vi "faultdia.vi"() -> ()   [LabVIEW 2018]
uses:
  <vilib>/Utility/file.llb/Read Delimited Spreadsheet (DBL).vi
panel:
  in  "选项卡控件":enum32{"分类训练", "状态监测", "故障诊断"}(tab)
  in  "隐藏层":dbl[](array[numeric])=[20.0, 20.0, 20.0]
  in  "残差值":dbl=1e-05
  in  "学习率":dbl=0.01
  in  "最大训练次数":dbl=1000.0
  out "训练完毕":bool
  out "导入完毕":bool
  in  "开始训练":bool
  in  "数据导入":bool
  in  "分类标签路径-output":path=path "E:/BIGzuoye2022/faultdig/gogoLabVIEW/faultdig/output.csv"
  in  "特征变量路径-input":path=path "E:/BIGzuoye2022/faultdig/gogoLabVIEW/faultdig/input.csv"
  out "总体分类结果\n Accuracy":dbl[](array[numeric])
  out "内阻偏大故障\n Accuracy":dbl[](array[numeric])
  out "SOC偏小故障\n Accuracy":dbl[](array[numeric])
  out "容量偏小故障\n Accuracy":dbl[](array[numeric])
  out "波形图":dbl[][](graph)
  out "all rows":dbl[][](array[numeric]) caption="特征变量查看"
  out "all rows 2":dbl[][](array[numeric]) caption="分类标签查看"
  in  "验证集-input":path=path "E:/BIGzuoye2022/faultdig/gogoLabVIEW/faultdig/variinput.csv"
  in  "验证集-output":path=path "E:/BIGzuoye2022/faultdig/gogoLabVIEW/faultdig/varioutput.csv"
  in  "继续监测":bool
  out "监测暂停":bool
  out "开始监测":bool
  in  "开始监测":bool
  in  "监测暂停":bool
  out "电压特征1实时监测":T1(graph)
  in  "Cell6连接":bool
  in  "Cell5连接":bool
  in  "Cell4连接":bool
  in  "Cell3连接":bool
  in  "Cell2连接":bool
  in  "Cell1连接":bool
  out "时间序列":dbl
  out "Cell1":dbl[](array[numeric])
  out "Cell2":dbl[](array[numeric])
  out "Cell3":dbl[](array[numeric])
  out "Cell4":dbl[](array[numeric])
  out "Cell5":dbl[](array[numeric])
  out "Cell6":dbl[](array[numeric])
  out "SOC实时监测":T1(graph)
  out "波形图表":T1(graph)
  out "随机生成特征变量":bool
  out "电池实时故障诊断":bool
  in  "电池实时故障诊断":bool
  out "电池监测时序":dbl
  in  "暂停诊断":bool
  in  "随机生成电池信息":bool
  out "电池正常1":bool[](array[boolean])
  out "内阻偏大故障1":bool[](array[boolean])
  out "SOC偏小故障1":bool[](array[boolean])
  out "容量偏小故障1":bool[](array[boolean])
  out "内阻偏大故障2":bool[](array[boolean])
  out "SOC偏小故障2":bool[](array[boolean])
  out "容量偏小故障2":bool[](array[boolean])
  out "电池正常2":bool[](array[boolean])
  out "内阻偏大故障3":bool[](array[boolean])
  out "SOC偏小故障3":bool[](array[boolean])
  out "容量偏小故障3":bool[](array[boolean])
  out "电池正常3":bool[](array[boolean])
  out "内阻偏大故障4":bool[](array[boolean])
  out "SOC偏小故障4":bool[](array[boolean])
  out "容量偏小故障4":bool[](array[boolean])
  out "电池正常4":bool[](array[boolean])
  out "内阻偏大故障5":bool[](array[boolean])
  out "SOC偏小故障5":bool[](array[boolean])
  out "容量偏小故障5":bool[](array[boolean])
  out "电池正常5":bool[](array[boolean])
  out "内阻偏大故障6":bool[](array[boolean])
  out "SOC偏小故障6":bool[](array[boolean])
  out "容量偏小故障6":bool[](array[boolean])
  out "电池正常6":bool[](array[boolean])
  in  "继续诊断":bool
  out "内阻偏大故障_rand":bool[](array[boolean])
  out "SOC偏小故障_rand":bool[](array[boolean])
  out "容量偏小故障_rand":bool[](array[boolean])
  out "电池正常_rand":bool[](array[boolean])
  out "随机生成特征变量 2":dbl[][](array[numeric])
  out "BP实际输出":dbl[][](array[numeric])
  out "诊断结果":dbl[][](array[numeric])
  # "默认：训练次数1000；学习率0.01；残差值0.00001；隐藏层[20,20,20].\n！！运行前修改文件路径！！"
  # "SOC\n\nSOC特征1\n\nSOC特征2\n\nSOC特征3\n\nSOC特征4\n\n电压特征1\n\n电压特征2\n\n电压特征3\n\n电压特征4"
  # "SOC\n\nSOC特征1\n\nSOC特征2\n\nSOC特征3\n\nSOC特征4\n\n电压特征1\n\n电压特征2\n\n电压特征3\n\n电压特征4"
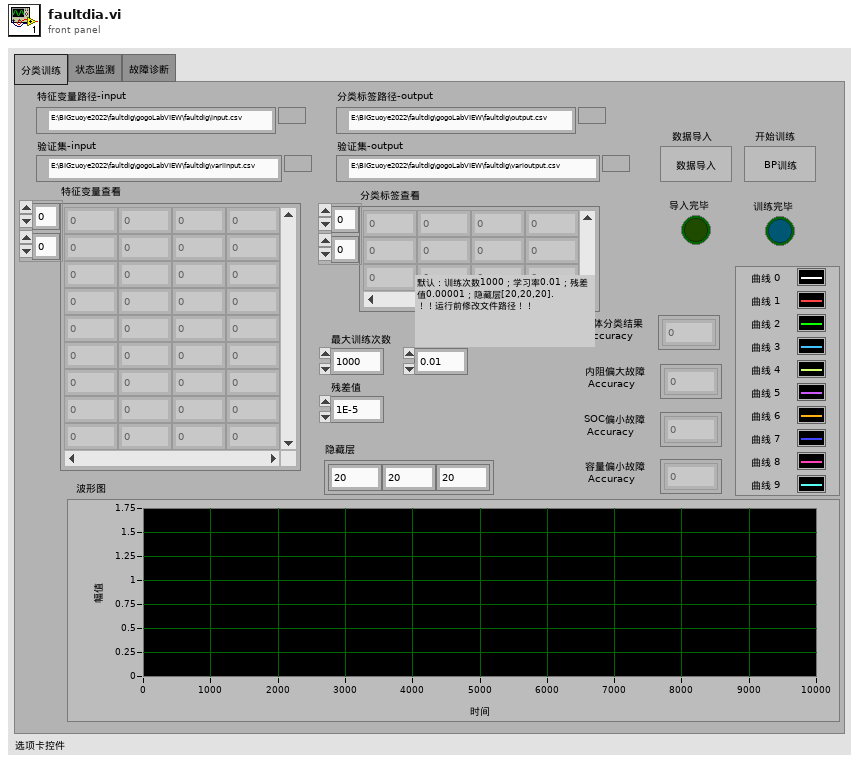
[diagram p1: front panel]
types:
  T1 = cluster{"Numeric":dbl, "Numeric":dbl, "Numeric":dbl, "Numeric":dbl, "Numeric":dbl, "Numeric":dbl}
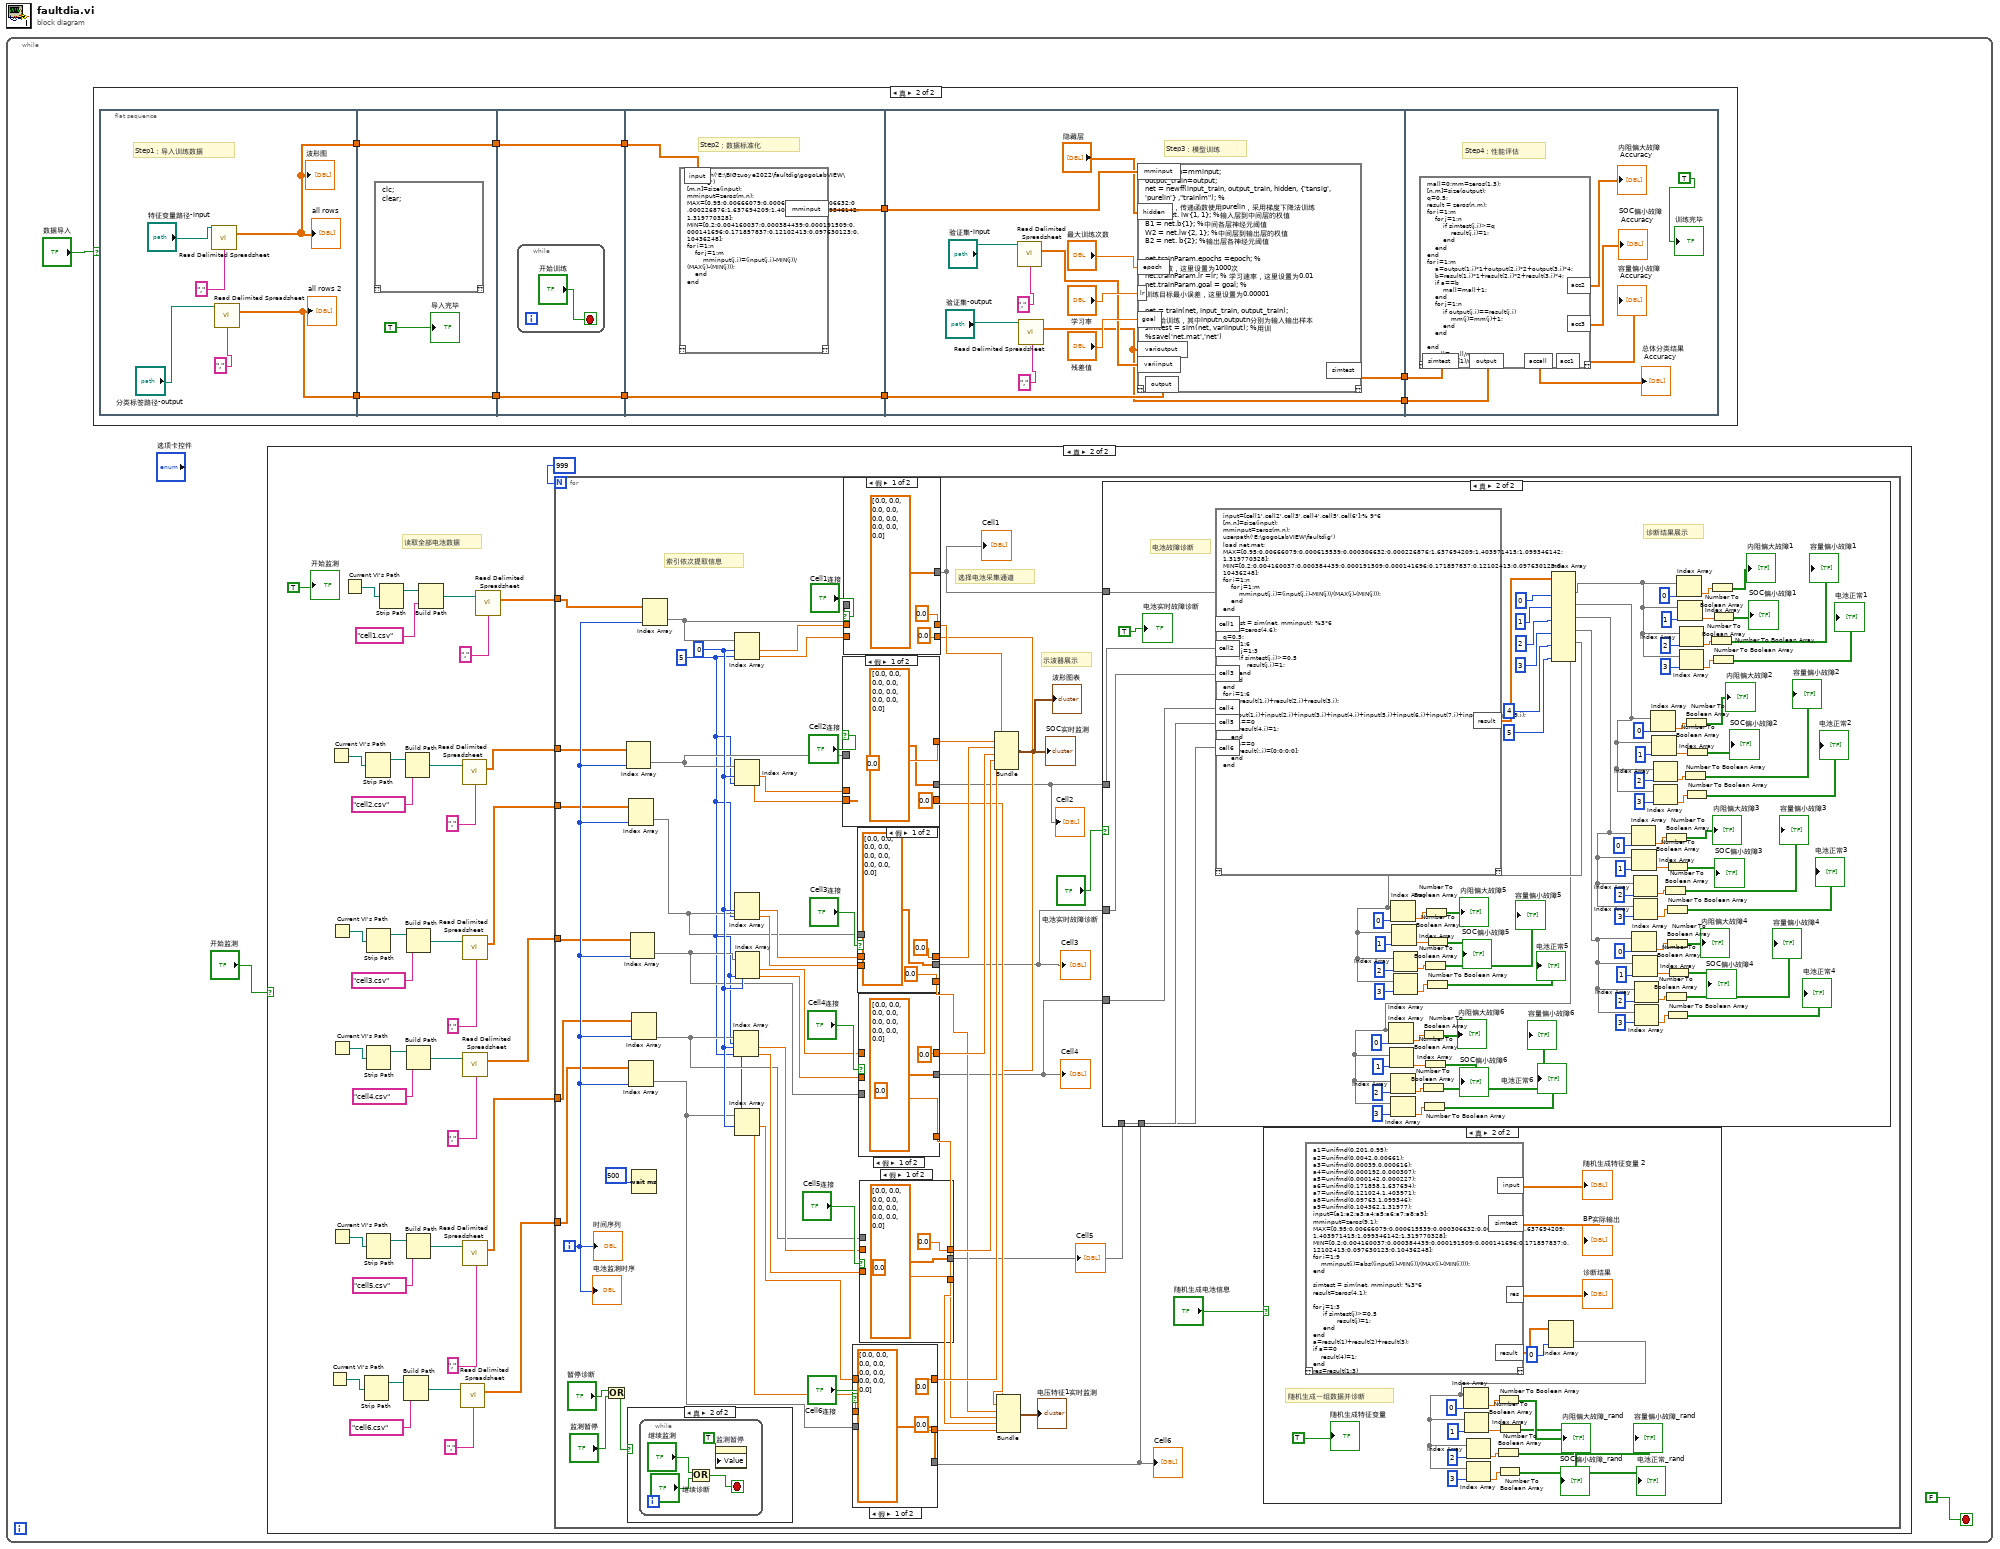
[diagram p0: block diagram]
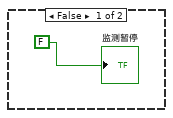
[diagram p11: hidden frame]
diagram:
  n1 = while {
    stop <- FALSE stop-if-true
    n2 = case shown="真" "数据导入" {
      frame False {
      }
      frame True {
        n3 = flat-sequence {
          tunnel: [w266] -> w262
          tunnel: [w265] -> w261
          tunnel: [w271] -> w260
          tunnel: w262 -> [w271]
          tunnel: w261 -> [w270]
          tunnel: [w270] -> w259
          tunnel: w260 -> [w273]
          tunnel: [w273] -> w258
          tunnel: w259 -> [w272]
          tunnel: [w272] -> w257
          tunnel: w258 -> [w277]
          tunnel: [w276] -> w256
          tunnel: [w275] -> w255
          tunnel: w257 -> [w275]
          tunnel: w256 -> [w290]
          tunnel: w255 -> [w288]
          tunnel: [w289] -> w254
          tunnel: [w278] -> w253
          tunnel: w254 -> [w297]
          tunnel: w253 -> [w291]
          frame #0 {
            # "Step1：导入训练数据"
            n4 = call-poly <vilib>:"Read Delimited Spreadsheet.vi"("file path (dialog if empty)"="特征变量路径-input", "delimiter (\\t)"=",") -> ("all rows"=w266:dbl[][])  [unwired: 8 in, 5 out]
            "all rows" <- w266
            "波形图" <- w266
            n5 = call-poly <vilib>:"Read Delimited Spreadsheet.vi"("file path (dialog if empty)"="分类标签路径-output", "delimiter (\\t)"=",") -> ("all rows"=w265:dbl[][])  [unwired: 8 in, 5 out]
            "all rows 2" <- w265
          }
          frame #1 {
            n6 = script code="clc;\nclear;"() -> ()  [unwired: 1 in, 1 out]
            "导入完毕" <- TRUE
          }
          frame #2 {
            n7 = while {
              stop <- "开始训练" stop-if-true
            }
          }
          frame #3 {
            # "Step2：数据标准化"
            n8 = script code="userpath('E:\\BIGzuoye2022\\faultdig\\gogoLabVIEW\\faultdig')\n[m,n]=size(input);\nmminput=zeros(m,n);\nMAX=[0.95;0.00666079;0.000615539;0.000306632;0.000226876;1.637694209;1.403971415;1.099346142;1.319770328];\nMIN=[0.2;0.004160037;0.000384439;0.000191509;0.000141696;0.171857837;0.12102413;0.097630123;0.10436248];\nfor i=1:n\n    for j=1:m\n        mminput(j,i)=(input(j,i)-MIN(j))/(MAX(j)-(MIN(j)));\n    end \nend"("input"=w277) -> ("mminput"=w276:dbl[][])  [unwired: 1 in, 1 out]
          }
          frame #4 {
            # "Step3：模型训练"
            n9 = call-poly <vilib>:"Read Delimited Spreadsheet.vi"("file path (dialog if empty)"="验证集-input", "delimiter (\\t)"=",") -> ("all rows"=w279:dbl[][])  [unwired: 8 in, 5 out]
            n10 = call-poly <vilib>:"Read Delimited Spreadsheet.vi"("file path (dialog if empty)"="验证集-output", "delimiter (\\t)"=",") -> ("all rows"=w278:dbl[][])  [unwired: 8 in, 5 out]
            n11 = script code="input_train=mminput;\noutput_train=output;\nnet = newff(input_train, output_train, hidden, {'tansig', 'purelin'} ,\"trainlm\"); % 建立模型，传递函数使用purelin，采用梯度下降法训练\nW1 = net. iw{1, 1}; %输入层到中间层的权值\nB1 = net.b{1}; %中间各层神经元阈值\nW2 = net.lw{2, 1}; %中间层到输出层的权值\nB2 = net. b{2}; %输出层各神经元阈值\n\nnet.trainParam.epochs =epoch; % 训练次数，这里设置为1000次\nnet.trainParam.lr =lr; % 学习速率，这里设置为0.01\nnet.trainParam.goal = goal; % 训练目标最小误差，这里设置为0.00001\n\nnet = train(net, input_train, output_train); %开始训练，其中inputn,outputn分别为输入输出样本\nsimtest = sim(net, variinput); %用训\n%save('net.mat','net')"("mminput"=w290, "output"=w288, "epoch"="最大训练次数", "lr"="学习率", "goal"="残差值", "hidden"="隐藏层", "varioutput"=w278, "variinput"=w279) -> ("simtest"=w289:dbl[][])  [unwired: 1 in, 1 out]
          }
          frame #5 {
            # "Step4：性能评估"
            n12 = script code="mall=0;mm=zeros(1,3);\n[n,m]=size(output);\nq=0.5;\nresult = zeros(n,m);\nfor i=1:m\n    for j=1:n\n        if simtest(j,i)>=q\n            result(j,i)=1;\n        end\n    end\nend\nfor i=1:m\n    a=output(1,i)*1+output(2,i)*2+output(3,i)*4;\n    b=result(1,i)*1+result(2,i)*2+result(3,i)*4;\n    if a==b\n        mall=mall+1;\n    end\n    for j=1:n\n        if output(j,i)==result(j,i)\n            mm(j)=mm(j)+1;\n        end\n    end\n    \nend\naccall=mall/m;\nacc1=mm(1)/m;\nacc2=mm(2)/m;\nacc3=mm(3)/m;"("output"=w291, "simtest"=w297) -> ("accall"=→"总体分类结果\n Accuracy":dbl[], "acc1"=→"容量偏小故障\n Accuracy":dbl[], "acc2"=→"内阻偏大故障\n Accuracy":dbl[], "acc3"=→"SOC偏小故障\n Accuracy":dbl[])  [unwired: 1 in, 1 out]
            "训练完毕" <- TRUE
          }
        }
      }
    }
    n13 = case shown="真" "开始监测" {
      frame False {
      }
      frame True {
        # "读取全部电池数据"
        n14 = Current VI's Path() -> (path=w30:path)
        n15 = Current VI's Path() -> (path=w10:path)
        n16 = Current VI's Path() -> (path=w15:path)
        n17 = Current VI's Path() -> (path=w20:path)
        n18 = Current VI's Path() -> (path=w25:path)
        n19 = Current VI's Path() -> (path=w41:path)
        n20 = Strip Path(path=w30) -> (stripped path=w31:path)  [unwired: 1 out]
        n21 = Strip Path(path=w10) -> (stripped path=w11:path)  [unwired: 1 out]
        n22 = Strip Path(path=w15) -> (stripped path=w16:path)  [unwired: 1 out]
        n23 = Strip Path(path=w20) -> (stripped path=w21:path)  [unwired: 1 out]
        n24 = Strip Path(path=w25) -> (stripped path=w26:path)  [unwired: 1 out]
        n25 = Strip Path(path=w41) -> (stripped path=w40:path)  [unwired: 1 out]
        n26 = Build Path(base path=w31, name or relative path="cell6.csv") -> (appended path=w33:path)
        n27 = Build Path(base path=w11, name or relative path="cell2.csv") -> (appended path=w13:path)
        n28 = Build Path(base path=w16, name or relative path="cell3.csv") -> (appended path=w18:path)
        n29 = Build Path(base path=w21, name or relative path="cell4.csv") -> (appended path=w23:path)
        n30 = Build Path(base path=w26, name or relative path="cell5.csv") -> (appended path=w28:path)
        n31 = Build Path(base path=w40, name or relative path="cell1.csv") -> (appended path=w38:path)
        n32 = call-poly <vilib>:"Read Delimited Spreadsheet.vi"("file path (dialog if empty)"=w33, "delimiter (\\t)"=",") -> ("all rows"=w5:dbl[][])  [unwired: 8 in, 5 out]
        n33 = call-poly <vilib>:"Read Delimited Spreadsheet.vi"("file path (dialog if empty)"=w13, "delimiter (\\t)"=",") -> ("all rows"=w9:dbl[][])  [unwired: 8 in, 5 out]
        n34 = call-poly <vilib>:"Read Delimited Spreadsheet.vi"("file path (dialog if empty)"=w18, "delimiter (\\t)"=",") -> ("all rows"=w8:dbl[][])  [unwired: 8 in, 5 out]
        n35 = call-poly <vilib>:"Read Delimited Spreadsheet.vi"("file path (dialog if empty)"=w23, "delimiter (\\t)"=",") -> ("all rows"=w7:dbl[][])  [unwired: 8 in, 5 out]
        n36 = call-poly <vilib>:"Read Delimited Spreadsheet.vi"("file path (dialog if empty)"=w28, "delimiter (\\t)"=",") -> ("all rows"=w6:dbl[][])  [unwired: 8 in, 5 out]
        n37 = call-poly <vilib>:"Read Delimited Spreadsheet.vi"("file path (dialog if empty)"=w38, "delimiter (\\t)"=",") -> ("all rows"=w35:dbl[][])  [unwired: 8 in, 5 out]
        n38 = for {
          N: 999 -> [_]
          tunnel: w35 -> [w58]
          tunnel: w9 -> [w57]
          tunnel: w8 -> [w56]
          tunnel: w7 -> [w55]
          tunnel: w6 -> [w54]
          tunnel: w5 -> [w53]
          i -> [w61]
          w59 = 5
          w99 = 0
          # "示波器展示"
          # "选择电池采集通道"
          # "索引依次提取信息"
          n39 = Or(x="暂停诊断", y="监测暂停") -> (x .or. y?=w44:bool)
          n40 = Index Array(array=w57, index (col)=w61) -> (element=w66:dbl[])  [unwired: 1 in]
          n41 = case shown="真" w44 {
            frame False {
              "监测暂停" <- FALSE
            }
            frame True {
              n42 = while {
                stop <- w249 stop-if-true
                n43 = Or(x="继续监测", y="继续诊断") -> (x .or. y?=w249:bool)
                n44 = property on="监测暂停" class="Bool (严格)"("Value"=TRUE) -> ()  [unwired: 2 in, 2 out]
              }
            }
          }
          n45 = Index Array(array=w56, index (col)=w61) -> (element=w65:dbl[])  [unwired: 1 in]
          n46 = Index Array(array=w53, index (col)=w61) -> (element=w62:dbl[])  [unwired: 1 in]
          n47 = Index Array(array=w55, index (col)=w61) -> (element=w64:dbl[])  [unwired: 1 in]
          n48 = Index Array(array=w54, index (col)=w61) -> (element=w63:dbl[])  [unwired: 1 in]
          n49 = Wait (ms)(milliseconds to wait=500) -> ()  [unwired: 1 out]
          n50 = Index Array(array=w58, index (col)=w61) -> (element=w67:dbl[])  [unwired: 1 in]
          n51 = Index Array(array=w63, index #1=w99, index #2=w59) -> (element #1=w84:dbl, element #2=w83:dbl)
          n52 = Index Array(array=w67, index #1=w99, index #2=w59) -> (element #1=w92:dbl, element #2=w91:dbl)
          n53 = Index Array(array=w66, index #1=w99, index #2=w59) -> (element #1=w90:dbl, element #2=w89:dbl)
          n54 = Index Array(array=w65, index #1=w99, index #2=w59) -> (element #1=w88:dbl, element #2=w87:dbl)
          n55 = Index Array(array=w62, index #1=w99, index #2=w59) -> (element #1=w82:dbl, element #2=w81:dbl)
          n56 = Index Array(array=w64, index #1=w99, index #2=w59) -> (element #1=w86:dbl, element #2=w85:dbl)
          n57 = case shown="假" "Cell2连接" {
            tunnel: w90 -> [_ w241]
            tunnel: w89 -> [_ w240]
            tunnel: [0.0 w241] -> w79
            tunnel: [0.0 w240] -> w70
            tunnel: [dbl[] [0.0, 0.0, 0.0, 0.0, 0.0, 0.0, 0.0, 0.0, 0.0] w239] -> w51
            tunnel: w66 -> [_ w239]
            frame False {
            }
            frame True {
            }
          }
          "Cell2" <- w51
          n58 = case shown="假" "Cell1连接" {
            tunnel: w92 -> [_ w247]
            tunnel: w91 -> [_ w246]
            tunnel: [0.0 w247] -> w80
            tunnel: [0.0 w246] -> w69
            tunnel: [dbl[] [0.0, 0.0, 0.0, 0.0, 0.0, 0.0, 0.0, 0.0, 0.0] w245] -> w52
            tunnel: w67 -> [_ w245]
            frame False {
            }
            frame True {
            }
          }
          "Cell1" <- w52
          n59 = case shown="假" "Cell6连接" {
            tunnel: w82 -> [_ w217]
            tunnel: w81 -> [_ w216]
            tunnel: [0.0 w217] -> w75
            tunnel: [0.0 w216] -> w74
            tunnel: [dbl[] [0.0, 0.0, 0.0, 0.0, 0.0, 0.0, 0.0, 0.0, 0.0] w215] -> w47
            tunnel: w62 -> [_ w215]
            frame False {
            }
            frame True {
            }
          }
          "Cell6" <- w47
          n60 = case shown="假" "Cell3连接" {
            tunnel: w88 -> [_ w235]
            tunnel: w87 -> [_ w234]
            tunnel: [0.0 w235] -> w78
            tunnel: [0.0 w234] -> w71
            tunnel: [dbl[] [0.0, 0.0, 0.0, 0.0, 0.0, 0.0, 0.0, 0.0, 0.0] w233] -> w50
            tunnel: w65 -> [_ w233]
            frame False {
            }
            frame True {
            }
          }
          "Cell3" <- w50
          n61 = case shown="假" "Cell4连接" {
            tunnel: w86 -> [_ w229]
            tunnel: w85 -> [_ w228]
            tunnel: [0.0 w229] -> w77
            tunnel: [0.0 w228] -> w72
            tunnel: [dbl[] [0.0, 0.0, 0.0, 0.0, 0.0, 0.0, 0.0, 0.0, 0.0] w227] -> w49
            tunnel: w64 -> [_ w227]
            frame False {
            }
            frame True {
            }
          }
          "Cell4" <- w49
          n62 = case shown="假" "Cell5连接" {
            tunnel: w84 -> [_ w223]
            tunnel: w83 -> [_ w222]
            tunnel: [0.0 w223] -> w76
            tunnel: [0.0 w222] -> w73
            tunnel: [dbl[] [0.0, 0.0, 0.0, 0.0, 0.0, 0.0, 0.0, 0.0, 0.0] w221] -> w48
            tunnel: w63 -> [_ w221]
            frame False {
            }
            frame True {
            }
          }
          "Cell5" <- w48
          n63 = Bundle("Numeric"=w80, "Numeric"=w79, "Numeric"=w78, "Numeric"=w77, "Numeric"=w76, "Numeric"=w75) -> (→"SOC实时监测" →"波形图表":T1)  [unwired: 1 in]
          n64 = Bundle("Numeric"=w69, "Numeric"=w70, "Numeric"=w71, "Numeric"=w72, "Numeric"=w73, "Numeric"=w74) -> (→"电压特征1实时监测":T1)  [unwired: 1 in]
          n65 = case shown="真" "电池实时故障诊断" {
            tunnel: w52 -> [_ w210]
            tunnel: w51 -> [_ w209]
            tunnel: w50 -> [_ w208]
            tunnel: w49 -> [_ w207]
            tunnel: w48 -> [_ w206]
            tunnel: w47 -> [_ w205]
            frame False {
            }
            frame True {
              # "诊断结果展示"
              # "电池故障诊断"
              n66 = script code="input=[cell1',cell2',cell3',cell4',cell5',cell6'];% 9*6\n[m,n]=size(input);\nmminput=zeros(m,n);\nuserpath('E:\\gogoLabVIEW\\faultdig')\nload net.mat;\nMAX=[0.95;0.00666079;0.000615539;0.000306632;0.000226876;1.637694209;1.403971415;1.099346142;1.319770328];\nMIN=[0.2;0.004160037;0.000384439;0.000191509;0.000141696;0.171857837;0.12102413;0.097630123;0.10436248];\nfor i=1:n\n    for j=1:m\n        mminput(j,i)=(input(j,i)-MIN(j))/(MAX(j)-(MIN(j)));\n    end \nend\n\nsimtest = sim(net, mminput); %3*6\nresult=zeros(4,6);\nq=0.5;\nfor i=1:6\n    for j=1:3\n        if simtest(j,i)>=0.5\n            result(j,i)=1;\n        end\n    end\nend\nfor i=1:6\n    a=result(1,i)+result(2,i)+result(3,i);\n    b=input(1,i)+input(2,i)+input(3,i)+input(4,i)+input(5,i)+input(6,i)+input(7,i)+input(8,i)+input(9,i);\n    if a==0\n        result(4,i)=1;\n    end\n    if b==0\n        result(:,i)=[0;0;0;0];\n    end\nend"("cell1"=w210, "cell2"=w209, "cell3"=w208, "cell4"=w207, "cell5"=w206, "cell6"=w205) -> ("result"=w204:dbl[][])  [unwired: 1 in, 1 out]
              n67 = Index Array(array=w204, index (col) #1=0, index (col) #2=1, index (col) #3=2, index (col) #4=3, index (col) #5=4, index (col) #6=5) -> (element #1=w189:dbl[], element #2=w124:dbl[], element #3=w123:dbl[], element #4=w122:dbl[], element #5=w121:dbl[], element #6=w120:dbl[])  [unwired: 6 in]
              n68 = Index Array(array=w120, index=0) -> (element=w133:dbl)
              n69 = Index Array(array=w120, index=1) -> (element=w134:dbl)
              n70 = Index Array(array=w121, index=0) -> (element=w145:dbl)
              n71 = Index Array(array=w120, index=2) -> (element=w135:dbl)
              n72 = Index Array(array=w120, index=3) -> (element=w136:dbl)
              n73 = Index Array(array=w121, index=1) -> (element=w146:dbl)
              n74 = Index Array(array=w121, index=2) -> (element=w147:dbl)
              n75 = Index Array(array=w121, index=3) -> (element=w148:dbl)
              n76 = Number To Boolean Array(number=w135) -> (Boolean array=→"容量偏小故障6":bool[])
              n77 = Number To Boolean Array(number=w133) -> (Boolean array=→"内阻偏大故障6":bool[])
              n78 = Number To Boolean Array(number=w136) -> (Boolean array=→"电池正常6":bool[])
              n79 = Number To Boolean Array(number=w147) -> (Boolean array=→"容量偏小故障5":bool[])
              n80 = Number To Boolean Array(number=w134) -> (Boolean array=→"SOC偏小故障6":bool[])
              n81 = Number To Boolean Array(number=w145) -> (Boolean array=→"内阻偏大故障5":bool[])
              n82 = Number To Boolean Array(number=w148) -> (Boolean array=→"电池正常5":bool[])
              n83 = Number To Boolean Array(number=w146) -> (Boolean array=→"SOC偏小故障5":bool[])
              n84 = Index Array(array=w123, index=0) -> (element=w169:dbl)
              n85 = Index Array(array=w123, index=1) -> (element=w170:dbl)
              n86 = Index Array(array=w122, index=0) -> (element=w157:dbl)
              n87 = Index Array(array=w122, index=1) -> (element=w158:dbl)
              n88 = Index Array(array=w123, index=2) -> (element=w171:dbl)
              n89 = Index Array(array=w123, index=3) -> (element=w172:dbl)
              n90 = Index Array(array=w122, index=2) -> (element=w159:dbl)
              n91 = Index Array(array=w122, index=3) -> (element=w160:dbl)
              n92 = Index Array(array=w124, index=0) -> (element=w181:dbl)
              n93 = Index Array(array=w124, index=1) -> (element=w182:dbl)
              n94 = Index Array(array=w124, index=2) -> (element=w183:dbl)
              n95 = Index Array(array=w124, index=3) -> (element=w184:dbl)
              n96 = Number To Boolean Array(number=w171) -> (Boolean array=→"容量偏小故障3":bool[])
              n97 = Number To Boolean Array(number=w169) -> (Boolean array=→"内阻偏大故障3":bool[])
              n98 = Number To Boolean Array(number=w159) -> (Boolean array=→"容量偏小故障4":bool[])
              n99 = Number To Boolean Array(number=w172) -> (Boolean array=→"电池正常3":bool[])
              n100 = Number To Boolean Array(number=w157) -> (Boolean array=→"内阻偏大故障4":bool[])
              n101 = Number To Boolean Array(number=w170) -> (Boolean array=→"SOC偏小故障3":bool[])
              n102 = Number To Boolean Array(number=w160) -> (Boolean array=→"电池正常4":bool[])
              n103 = Number To Boolean Array(number=w158) -> (Boolean array=→"SOC偏小故障4":bool[])
              n104 = Index Array(array=w189, index=0) -> (element=w194:dbl)
              n105 = Index Array(array=w189, index=1) -> (element=w195:dbl)
              n106 = Index Array(array=w189, index=2) -> (element=w196:dbl)
              n107 = Index Array(array=w189, index=3) -> (element=w197:dbl)
              n108 = Number To Boolean Array(number=w183) -> (Boolean array=→"容量偏小故障2":bool[])
              n109 = Number To Boolean Array(number=w181) -> (Boolean array=→"内阻偏大故障2":bool[])
              n110 = Number To Boolean Array(number=w184) -> (Boolean array=→"电池正常2":bool[])
              n111 = Number To Boolean Array(number=w182) -> (Boolean array=→"SOC偏小故障2":bool[])
              n112 = Number To Boolean Array(number=w196) -> (Boolean array=→"容量偏小故障1":bool[])
              n113 = Number To Boolean Array(number=w194) -> (Boolean array=→"内阻偏大故障1":bool[])
              n114 = Number To Boolean Array(number=w197) -> (Boolean array=→"电池正常1":bool[])
              n115 = Number To Boolean Array(number=w195) -> (Boolean array=→"SOC偏小故障1":bool[])
              "电池实时故障诊断" <- TRUE
            }
          }
          n116 = case shown="真" "随机生成电池信息" {
            frame False {
            }
            frame True {
              # "随机生成一组数据并诊断"
              n117 = script code="a1=unifrnd(0.201,0.95);\na2=unifrnd(0.0042,0.00661);\na3=unifrnd(0.00039,0.000616);\na4=unifrnd(0.000192,0.000307);\na5=unifrnd(0.000142,0.000227);\na6=unifrnd(0.171858,1.637694);\na7=unifrnd(0.121024,1.403971);\na8=unifrnd(0.09763,1.099346);\na9=unifrnd(0.104362,1.31977);\ninput=[a1;a2;a3;a4;a5;a6;a7;a8;a9];\nmminput=zeros(9,1);\nMAX=[0.95;0.00666079;0.000615539;0.000306632;0.000226876;1.637694209;1.403971415;1.099346142;1.319770328];\nMIN=[0.2;0.004160037;0.000384439;0.000191509;0.000141696;0.171857837;0.12102413;0.097630123;0.10436248];\nfor i=1:9\n    mminput(i)=abs((input(i)-MIN(i))/(MAX(i)-(MIN(i))));\nend\n\nsimtest = sim(net, mminput); %3*6\nresult=zeros(4,1);\n\nfor j=1:3\n     if simtest(j)>=0.5\n            result(j)=1;\n     end\nend\na=result(1)+result(2)+result(3);\nif a==0\n    result(4)=1;\nend\nres=result(1:3)"() -> ("input"=→"随机生成特征变量 2":dbl[][], "simtest"=→"BP实际输出":dbl[][], "result"=w103:dbl[][], "res"=→"诊断结果":dbl[][])  [unwired: 1 in, 1 out]
              n118 = Index Array(array=w103, index (col)=0) -> (element=w101:dbl[])  [unwired: 1 in]
              n119 = Index Array(array=w101, index=0) -> (element=w116:dbl)
              n120 = Index Array(array=w101, index=1) -> (element=w117:dbl)
              n121 = Index Array(array=w101, index=2) -> (element=w118:dbl)
              n122 = Index Array(array=w101, index=3) -> (element=w119:dbl)
              n123 = Number To Boolean Array(number=w118) -> (Boolean array=→"容量偏小故障_rand":bool[])
              n124 = Number To Boolean Array(number=w116) -> (Boolean array=→"内阻偏大故障_rand":bool[])
              n125 = Number To Boolean Array(number=w119) -> (Boolean array=→"电池正常_rand":bool[])
              n126 = Number To Boolean Array(number=w117) -> (Boolean array=→"SOC偏小故障_rand":bool[])
              "随机生成特征变量" <- TRUE
            }
          }
          "时间序列" <- w61
          "电池监测时序" <- w61
        }
        "开始监测" <- TRUE
      }
    }
  }
